vi "Save Data.vi"(8 "error in (no error)":errorcluster, 11 "Pulse Driver in":refnum<class "Pulse Driver.lvclass">) -> (0 "error out":errorcluster, 1 "Finished":bool, 2 "Current read position":i32, 3 "Pulse Driver out":refnum<class "Pulse Driver.lvclass">)   [LabVIEW 2016, in "Pulse Driver.lvclass"]
uses:
  Pulse Driver.lvclass
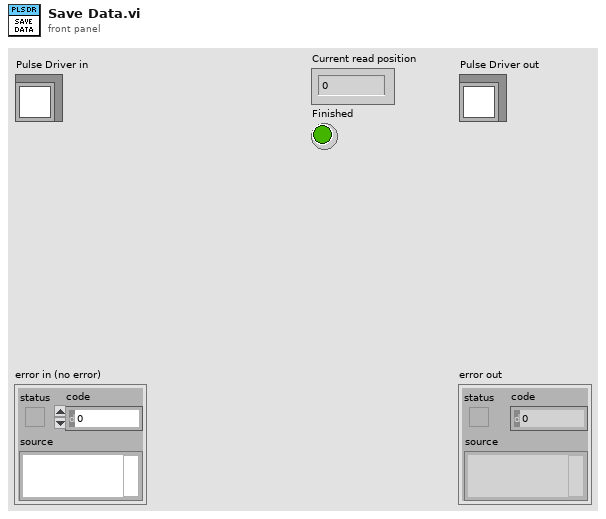
[diagram p1: front panel]
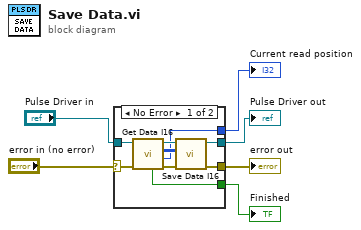
[diagram p0: block diagram]
diagram:
  n1 = case shown="No Error" "error in (no error)" {
    selector: "error in (no error)" -> [w13 w17]
    tunnel: [w12 w17] -> w5
    tunnel: [w10 w16] -> w3
    tunnel: "Pulse Driver in" -> [w11 w16]
    tunnel: [w8 _] -> w2
    tunnel: [w7 _] -> w1
    frame No Error {
      n2 = call-dynamic "Get Data I16.vi"("error in (no error)"=w13, "Pulse Driver in"=w11) -> ("error out"=w14:errorcluster, "Current read position"=w8:i32, "Data out"=w9:i16[][], "Pulse Driver out"=w15:refnum<class "Pulse Driver.lvclass">, "Finished"=w7:bool)  [unwired: 5 in]
      n3 = call-dynamic "Save Data I16.vi"("error in (no error)"=w14, "Data"=w9, "Pulse Driver in"=w15) -> ("error out"=w12:errorcluster, "Pulse Driver out"=w10:refnum<class "Pulse Driver.lvclass">)  [unwired: 7 in]
    }
    frame Error {
    }
  }
  "error out" <- w5
  "Pulse Driver out" <- w3
  "Current read position" <- w2
  "Finished" <- w1
